vi "MultiDiagramStructureToJson.vi"(6 "Component Idx":i32, 7 "Relative Bounds":cluster{"x":i32, "y":i32, "w":i32, "h":i32}, 8 "error in (no error)":errorcluster, 9 "Origin Path":path, 10 "Current Path":path, 11 "MultiDiagramStructure in":refnum<vi>) -> (0 "error out":errorcluster, 2 "JSON":string)   [LabVIEW 2017]
doc: "Creates a JSON for a Multidiagram Structure"
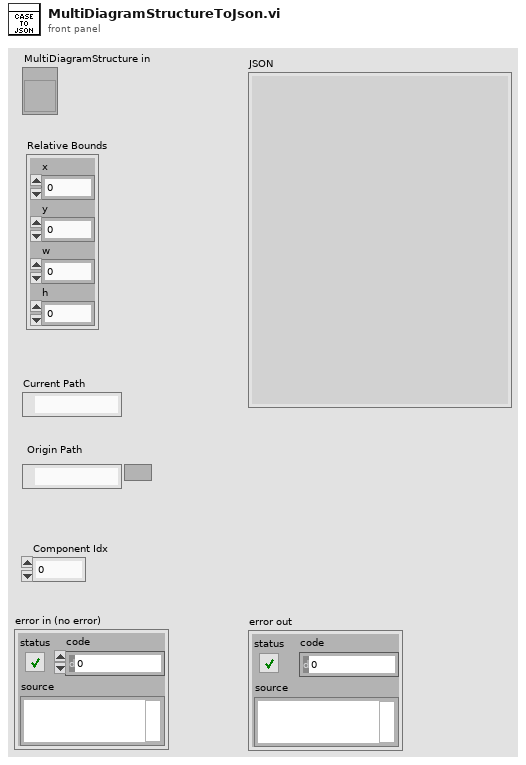
[diagram p1: front panel]
types:
  T1 = typedef "LVRectTypeDef.ctl" = cluster{"Left":i16, "Top":i16, "Right":i16, "Bottom":i16}
  T2 = typedef "imagedata.ctl" = cluster{"image type":i32, "image depth":i32, "image":u8[], "mask":u8[], "colors":u32[], "Rectangle":cluster{"left":i16, "top":i16, "right":i16, "bottom":i16}}
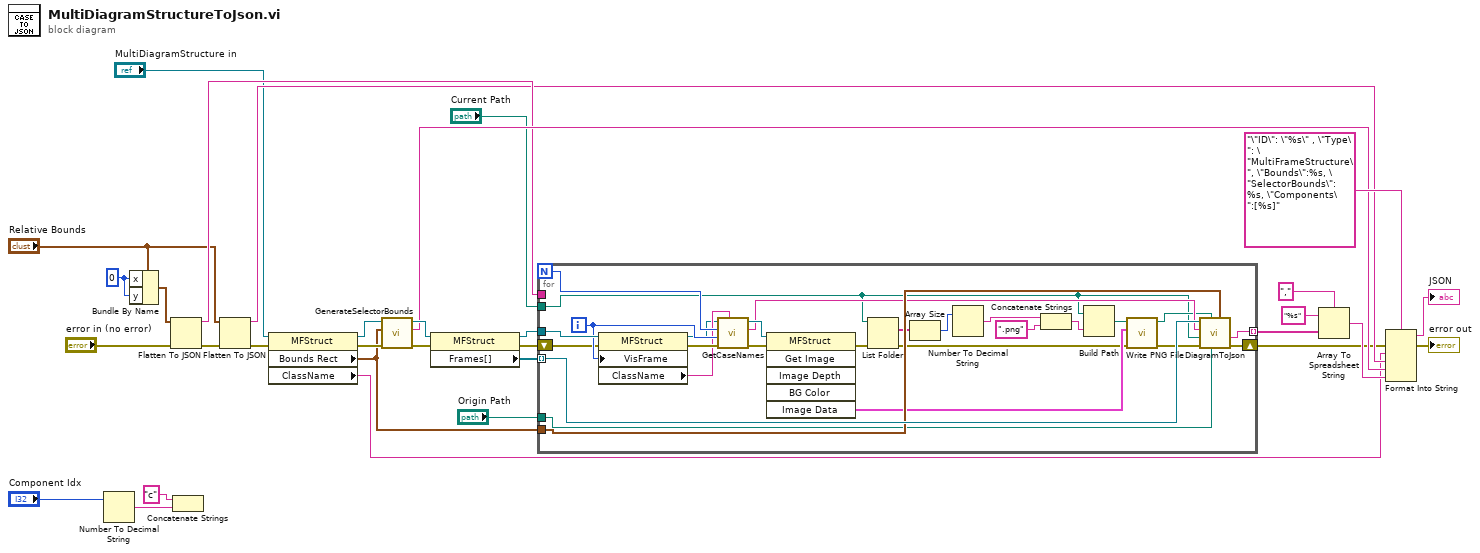
[diagram p0: block diagram]
diagram:
  w10 = 0 ("x")
  n1 = Number To Decimal String(number="Component Idx") -> (decimal integer string=w28:string)  [unwired: 1 in]
  n2 = Bundle By Name(cluster="Relative Bounds", "x"=w10, "y"=w10) -> (w22:cluster{"x":i32, "y":i32, "w":i32, "h":i32})
  n3 = Flatten To JSON(anything=w22, error in (no error)="error in (no error)") -> (JSON string=w21:string, 11:w8:errorcluster)  [unwired: 1 in]
  n4 = Concatenate Strings("c" ("string"), w28) -> ()  [unwired: 1 out]
  n5 = Flatten To JSON(anything="Relative Bounds", error in (no error)=w8) -> (JSON string=w16:string, 11:w7:errorcluster)  [unwired: 1 in]
  n6 = property class="MFStruct"(reference="MultiDiagramStructure in", error in=w7) -> (reference out=w13:refnum<vi>, error out=w9:errorcluster, "Bounds Rect"=w5:T1, "ClassName"=w4:string)
  n7 = call "GenerateSelectorBounds.vi"("error in (no error)"=w9, "Master Bounds Rect"=w5, "MultiFrameStructure in"=w13) -> ("error out"=w12:errorcluster, "JSON string"=w25:string, "reference out"=w29:refnum<vi>)  [unwired: 6 in]
  n8 = property class="MFStruct"(reference=w29, error in=w12) -> (reference out=w23:refnum<vi>, error out=w6:errorcluster, "Frames[]"=w24:refnum<vi>[])
  n9 = for {
    N -> [w53]
    tunnel: w24 -> [w58] mode=indexing
    tunnel: w23 -> [w59]
    tunnel: "Current Path" -> [w40]
    tunnel: w5 -> [w55]
    tunnel: "Origin Path" -> [w54]
    tunnel: w21 -> [_]
    tunnel: [w42] -> w18 mode=indexing
    shift-right: [w43] -> w15
    shift-left: w6 -> [w46]
    i -> [w56]
    n10 = property class="MFStruct"(reference=w59, error in=w46, "VisFrame"=w56) -> (reference out=w50:refnum<vi>, error out=w57:errorcluster, "ClassName"=w51:string)
    n11 = call "GetCaseNames.vi"("ClassName"=w51, "error in (no error)"=w57, "DiagramIndex"=w56, "DiagramCount"=w53, "MultiFrameStructure in"=w50) -> ("error out"=w48:errorcluster, "String"=w45:string, "MultiFrameStructure out"=w49:refnum<vi>)  [unwired: 4 in]
    n12 = invoke class="MFStruct" method="Get Image"(reference=w49, error in=w48) -> (error out=w34:errorcluster, "Image Data"=w47:T2)  [unwired: 4 in, 4 out]
    n13 = List Folder(path=w40, error in=w34) -> (filenames=w39:string[], error out=w33:errorcluster)  [unwired: 2 in, 2 out]
    n14 = Array Size(array=w39) -> (size(s)=w38:i32)
    n15 = Number To Decimal String(number=w38) -> (decimal integer string=w37:string)  [unwired: 1 in]
    n16 = Concatenate Strings(w37, ".png" ("string")) -> (w35:string)
    n17 = Build Path(base path=w40, name or relative path=w35) -> (appended path=w41:path)
    n18 = call <vilib>:"Write PNG File.vi"("error in (no error)"=w33, "image data"=w47, "path to PNG file"=w41) -> ("error out"=w52:errorcluster, "path"=w44:path)  [unwired: 7 in]
    n19 = call "DiagramToJson.vi"("Owner Bounds"=w55, "Origin Path"=w54, "Image Path"=w44, "error in (no error)"=w52, "Current Path"=w40, "ID"=w45, "GObj in"=w58) -> ("error out"=w43:errorcluster, "JSON (out)"=w42:string)  [unwired: 2 in, 1 out]
  }
  n20 = Array To Spreadsheet String(delimiter (Tab)=",", array=w18, 3:"%s" ("format string")) -> (spreadsheet string=w17:string)
  n21 = Format Into String(format string="\"ID\": \"%s\" , \"Type\": \"MultiFrameStructure\", \"Bounds\":%s, \"SelectorBounds\": %s, \"Components\":[%s]", error in=w15, w4, w16, w25, w17) -> (resulting string=→"JSON":string, error out=→"error out":errorcluster)  [unwired: 1 in]
